vi "write_params.vi"(8 "error in (no error)":errorcluster, 10 "params":T1={"base_estimator"="None", "n_estimators"=10.0, "max_samples"={"max_samples_type"="float", "max_samples_float"=1.0, "max_samples_int"=0.0}, "max_features"={"max_features_type"="float", "max_features_float"=1.0, "max_features_int"=0.0}, "bootstrap"=TRUE, "bootstrap_features"=FALSE, "oob_score"=FALSE, "warm_start"=FALSE, "n_jobs"=1.0, "random_state"=0.0, "verbose"=0.0}, 11 "BaggingClassifier in":refnum<class "BaggingClassifier.lvclass">) -> (0 "error out":errorcluster, 3 "BaggingClassifier out":refnum<class "BaggingClassifier.lvclass">)   [LabVIEW 2020, in "BaggingClassifier.lvclass"]
uses:
  BaggingClassifier.lvclass
  Controls/bagging_classifier_params.ctl
  BaggingClassifier.lvclass/BaggingClassifier.ctl
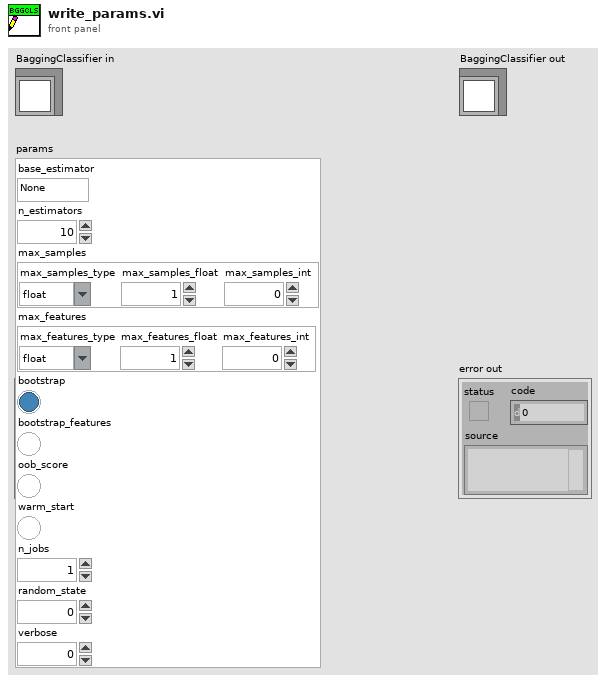
[diagram p1: front panel]
types:
  T1 = typedef "bagging_classifier_params.ctl" = cluster{"base_estimator":string, "n_estimators":dbl, "max_samples":cluster{"max_samples_type":string, "max_samples_float":dbl, "max_samples_int":dbl}, "max_features":cluster{"max_features_type":string, "max_features_float":dbl, "max_features_int":dbl}, "bootstrap":bool, "bootstrap_features":bool, "oob_score":bool, "warm_start":bool, "n_jobs":dbl, "random_state":dbl, "verbose":dbl}
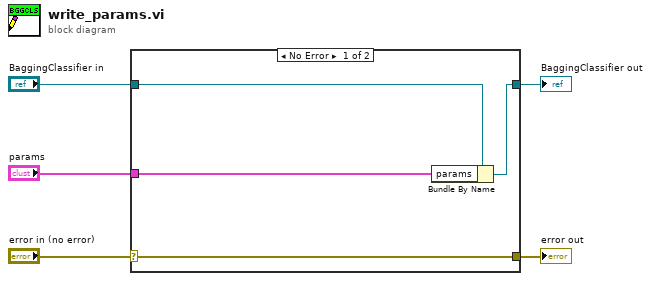
[diagram p0: block diagram]
diagram:
  n1 = case shown="No Error" "error in (no error)" {
    selector: "error in (no error)" -> [w9 w10]
    tunnel: [w9 w10] -> w4
    tunnel: [w7 w11] -> w2
    tunnel: "BaggingClassifier in" -> [w8 w11]
    tunnel: "params" -> [w6 _]
    frame No Error {
      n2 = Bundle By Name(cluster=w8, "params"=w6) -> (w7:refnum<class "BaggingClassifier.lvclass">)
    }
    frame Error {
    }
  }
  "error out" <- w4
  "BaggingClassifier out" <- w2
